vi "Moving Average  and AI Filter testing.vi"() -> ()   [LabVIEW 2009]
uses:
  Controls/SLL DE DAQ Parameters LV2Global Options.ctl
  <vilib>/Analysis/3filter.llb/Butterworth Filter (DBL).vi
  <vilib>/measure/NI_MABase.lvlib
  <vilib>/Analysis/NI_AALBase.lvlib
panel:
  out "size(s)":i32
  in  "stop":bool
  in  "noise (rms)":dbl=0.05 step=0.05
  in  "Window Size":i32=3
  out "Waveform Chart":waveform(dbl)[](graph)
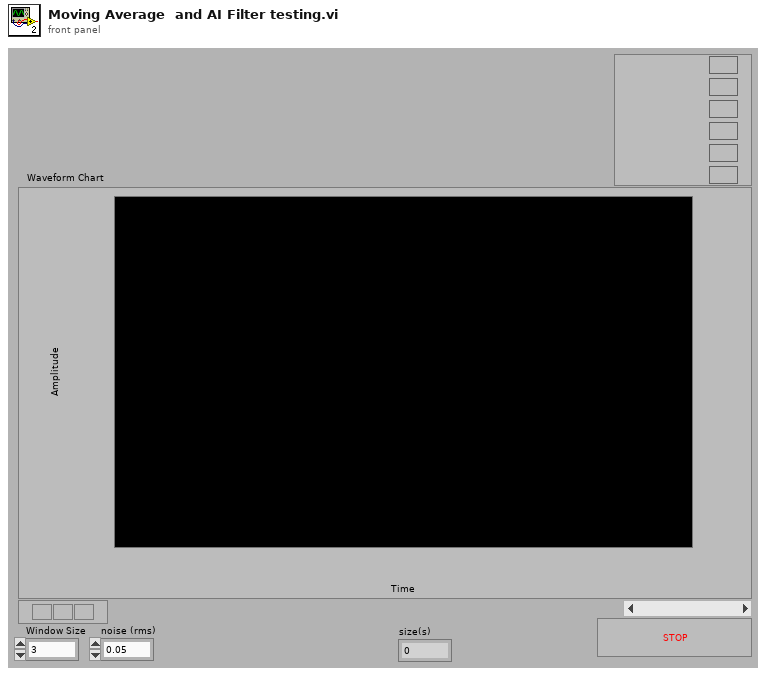
[diagram p1: front panel]
types:
  T1 = typedef "SLL DE DAQ Parameters LV2Global Options.ctl" = enum16{"Read", "Write"}
  T2 = enum32{"Lowpass", "Highpass", "Bandpass", "Bandstop"}
  T3 = typedef "SLL DE DAQ Engine Parameters.ctl" = cluster{"Enable Engines":cluster{"AI Enable":bool, "AO Enable":bool, "DI Enable":bool, "DO Enable":bool}, "DAQ Control Type":cluster{"Analog Input":enum16{"Finite", "Continuous", "Driver"}, "Analog Output":enum16{"Finite", "Continuous", "Driver"}, "Digital Input":enum16{"Finite", "Continuous", "Driver"}, "Digital Output":enum16{"Finite", "Continuous", "Driver"}}, "DAQ Parameters":cluster{"AI Sampling Rate (Samples/Sec)":dbl, "MvgAVG Window Size (# of Points)":i32, "Enable Filter":bool, "Enable MvgAVG":bool, "Circular Buffer Size (Sec)":dbl, "AO Sampling Rate (Samples/Sec)":dbl, "Graph Update Rate (Samples/Sec)":dbl, "File Logging Rate (Samples/Sec)":i32}, "AO Safe Values":cluster{"Analog Outputs Name":T4, "Analog Outputs Safe Value":dbl}[], "DO Safe Values":cluster{"Digital Outputs Name":T5, "Digital Outputs Safe Value":bool}[], "DO Interconnected Lines":cluster{"First DO Line":string, "Second DO Line":string}[], "AI Channels Unit":cluster{"Channel Name":T6, "Channel Type":T7}[], "Units Information":cluster{"Channel Type":T7, "Unit Text":string, "Maximum":dbl, "Minmum":dbl, "Increments":dbl}[]}
  T4 = typedef "SLL DE List of Analog Outputs.ctl" = enum16{"PP01TS", "PP02TS", "PP03TS"}
  T5 = typedef "SLL DE List of Digital Outputs.ctl" = enum16{"SL01TS", "SL02TS", "SV01TS", "SV02TS", "SV03TS", "SV04TS", "SV05TS", "SV06TS", "SV07TS", "SV08TS", "SV09TS", "SV10TS", "SV11TS", "SV12TS", "SV13TS", "SV14TS", "SV15TS", "SV16TS", "SV17TS", "SV18TS", "SV19TS", "SV20TS", "SV21TS", "SV22TS", "SV23TS", "SV24TS", "SV25TS", "SV26TS", "SV27TS", "SV28TS", "SV29TS", "SV30TS", "SV31TS", "SV32TS", "SV33TS", "SV34TS", "SV35TS", "SV36TS", "SV37TS", "SV38TS", "SV39TS", "SV40TS", "SV41TS", "SV42TS", "SV43TS", "SV44TS", "SV45TS", "SV46TS", "SV47TS", "SV48TS", "SV49TS", "SV50TS", "SV51TS", "SV52TS", "SV53TS", "SV54TS", "SV55TS", "SV56TS", "SV57TS"}
  T6 = typedef "SLL DE List of Analog Inputs.ctl" = enum16{"FM01TS", "FM02TS", "FM03TS", "FM04TS", "FM05TS", "PC01TS", "PC02TS", "PC03TS", "PT01TS", "PT02TS", "PT03TS", "PT04TS", "PT05TS", "PT06TS", "ST01TS", "TC01TS", "TC02TS", "TC03TS", "TT01TS"}
  T7 = typedef "SLL DE List of AI Channel Type.ctl" = enum16{"Pressure", "Flow", "Temperature", "Time Scale", "Voltage", "Current", "Frequency", "Sound", "Speed", "Torque", "Distance", "Channel Type 1", "Channel Type 2", "Channel Type 3"}
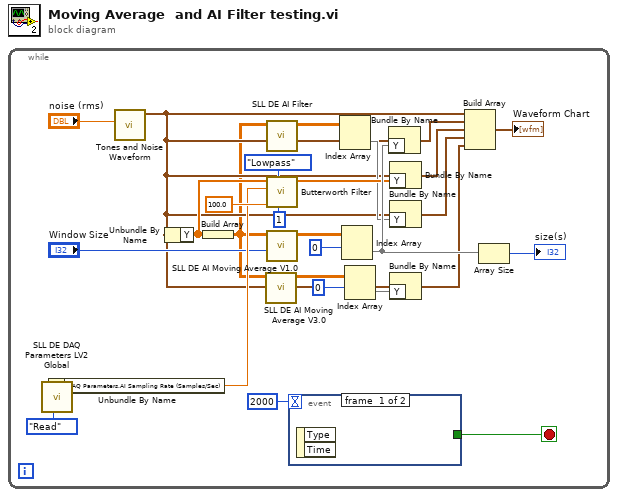
[diagram p0: block diagram]
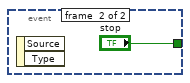
[diagram p2: hidden frame]
diagram:
  n1 = while {
    stop <- w25 stop-if-true
    n2 = call "SLL DE DAQ Parameters LV2 Global.vi"("Option"=SLL_DE_DAQ_Parameters_LV2Global_Options."Read") -> ("Global Info"=w14:T3)  [unwired: 9 in, 1 out]
    n3 = Unbundle By Name(w14) -> ("DAQ Parameters.AI Sampling Rate (Samples/Sec)"=w13:dbl)
    n4 = call <vilib>:"Tones and Noise Waveform.vi"("noise (rms)"="noise (rms)") -> ("signal out"=w3:waveform(dbl))  [unwired: 6 in, 4 out]
    n5 = Unbundle By Name(w3) -> ("Y"=w5:dbl[])
    n6 = Build Array(w5) -> (w2:dbl[][])
    n7 = call "SLL DE AI Moving Average V3.0.vi"("Input Array"=w2) -> ("Averaged Array"=w1:dbl[][])  [unwired: 9 in, 1 out]
    n8 = call "SLL DE AI Filter.vi"("Raw Data"=w2) -> ("Filtered Avg Data"=w11:dbl[][])  [unwired: 9 in, 1 out]
    n9 = call-poly <vilib>:"Butterworth Filter.vi"("order"=1, "filter type"=T2."Lowpass", "low cutoff freq: fl"=100.0, "sampling freq: fs"=w13, "X"=w5) -> ("Filtered X"=w12:dbl[])  [unwired: 3 in, 1 out]
    n10 = call "SLL DE AI Moving Average V1.0.vi"("Window Size"="Window Size", "Array"=w2) -> ("Average Array"=w24:dbl[][])  [unwired: 8 in, 1 out]
    n11 = event shown="[1] \"stop\": Value Change" {
      selector: _ -> [_ _]
      dyn-events: _ -> [_ _]
      timeout: 2000 -> [_ _]
      tunnel: [_ "stop"] -> w25
      event #0 {
        n12 = event-data() -> ()  [unwired: 3 out]
      }
      event #1 {
        n13 = event-data() -> ()  [unwired: 3 out]
      }
    }
    n14 = Index Array(array=w11) -> (element=w9:dbl[])  [unwired: 2 in]
    n15 = Index Array(array=w24, index (row)=0 ("disabled index (col)")) -> (element=w22:dbl[])  [unwired: 1 in]
    n16 = Index Array(array=w1, index (row)=0 ("disabled index (col)")) -> (element=w7:dbl[])  [unwired: 1 in]
    n17 = Bundle By Name(cluster=w3, "Y"=w22) -> (w23:waveform(dbl))
    n18 = Bundle By Name(cluster=w3, "Y"=w12) -> (w19:waveform(dbl))
    n19 = Bundle By Name(cluster=w3, "Y"=w9) -> (w10:waveform(dbl))
    n20 = Bundle By Name(cluster=w3, "Y"=w7) -> (w6:waveform(dbl))
    n21 = Build Array(w3, w23, w19, w10, w6) -> (→"Waveform Chart":waveform(dbl)[])
    n22 = Array Size(array=w22) -> (size(s)=→"size(s)":i32)
  }
